vi "Warfortheworlds.vi"() -> ()   [LabVIEW 2021]
panel:
  out "ReadComplete":bool
  out "CountComplete":bool
  out "number":i32
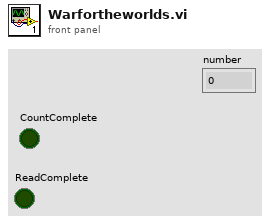
[diagram p1: front panel]
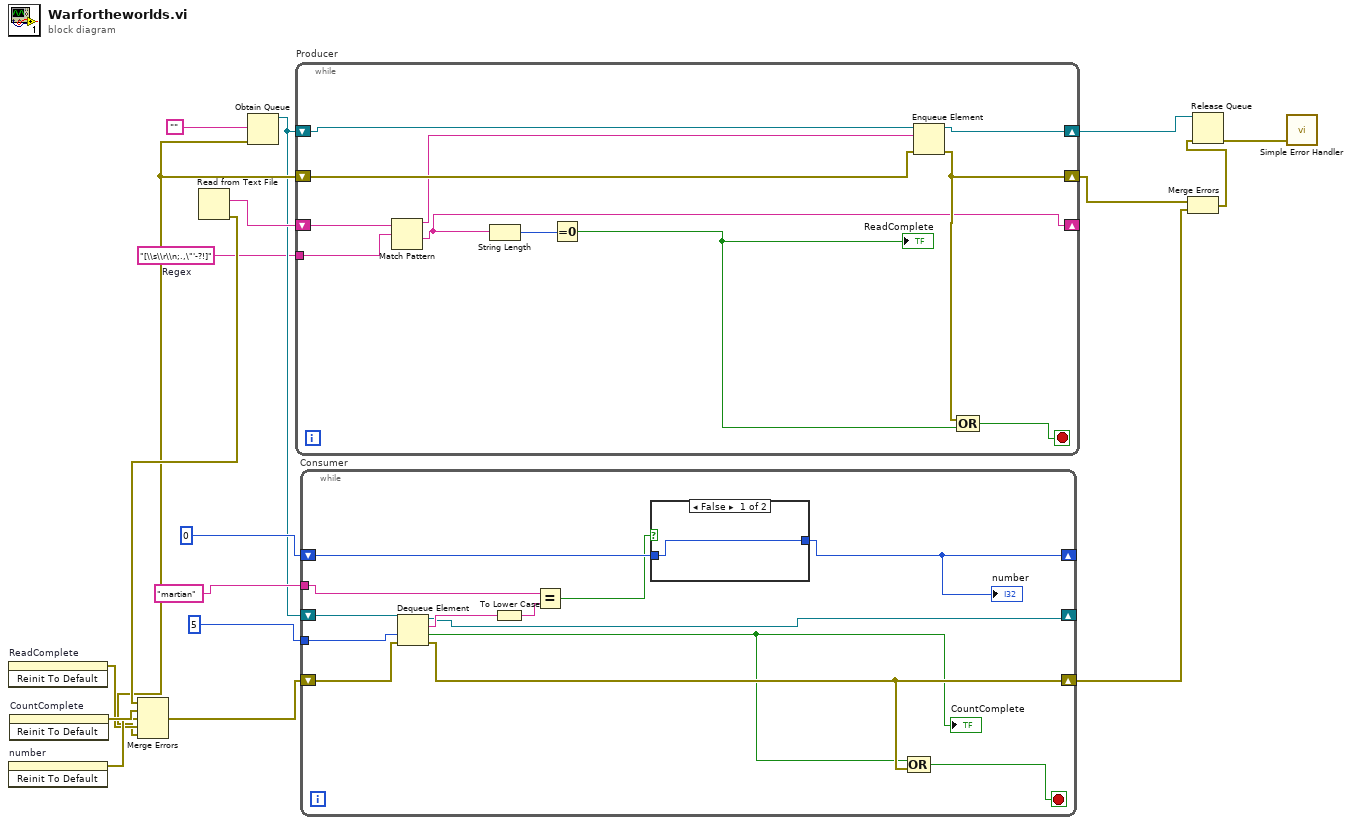
[diagram p0: block diagram]
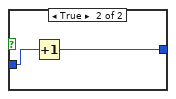
[diagram p2: hidden frame]
diagram:
  w1 = "[\\s\\r\\n;.,\"'-?!]"  # Regex
  n1 = invoke on="ReadComplete" class="Bool (strict)" method="Reinit To Default"() -> (error out=w7:errorcluster)  [unwired: 3 in, 2 out]
  n2 = invoke on="number" class="DigNum (strict)" method="Reinit To Default"() -> (error out=w8:errorcluster)  [unwired: 3 in, 2 out]
  n3 = invoke on="CountComplete" class="Bool (strict)" method="Reinit To Default"() -> (error out=w9:errorcluster)  [unwired: 3 in, 2 out]
  n4 = Read from Text File() -> (text=w17:string, error out=w6:errorcluster)  [unwired: 4 in, 2 out]
  n5 = Obtain Queue(element data type="") -> (queue out=w3:refnum<queue>, error out=w5:errorcluster)  [unwired: 4 in, 1 out]
  n6 = Merge Errors(w6, w9, w8, w7, w5) -> (w4:errorcluster)
  n7 = while "Producer" {
    shift-right: [w27] -> w14
    shift-left: w3 -> [w29]
    shift-right: [w23] -> w15
    shift-left: w5 -> [w28]
    shift-right: [w22] -> _
    shift-left: w17 -> [w26]
    tunnel: w1 -> [w19]
    stop <- w21 stop-if-true
    n8 = Match Pattern(string=w26, regular expression=w19) -> (before substring=w20:string, after substring=w22:string)  [unwired: 1 in, 2 out]
    n9 = String Length(string=w22) -> (length=w25:i32)
    n10 = Equal To 0?(x=w25) -> (x = 0?=w24:bool)
    "ReadComplete" <- w24
    n11 = Enqueue Element(queue=w29, element=w20, error in (no error)=w28) -> (queue out=w27:refnum<queue>, error out=w23:errorcluster)  [unwired: 1 in, 1 out]
    n12 = Compound Arithmetic op=OR(w23, w24) -> (w21:bool)
  }
  n13 = while "Consumer" {
    shift-right: [w32] -> _
    shift-left: 0 -> [w33]
    shift-right: [w31] -> _
    shift-left: w3 -> [w40]
    shift-right: [w39] -> w2
    shift-left: w4 -> [w42]
    tunnel: "martian" -> [w34]
    tunnel: 5 -> [w41]
    stop <- w38 stop-if-true
    n14 = Dequeue Element(queue=w40, timeout in ms (-1)=w41, error in (no error)=w42) -> (queue out=w31:refnum<queue>, element=w35:string, timed out?=w37:bool, error out=w39:errorcluster)
    "CountComplete" <- w37
    n15 = To Lower Case(string=w35) -> (all lower case string=w36:string)
    n16 = Equal?(x=w34, y=w36) -> (x = y?=w30:bool)
    n17 = case shown="False" w30 {
      tunnel: w33 -> [w43 w45]
      tunnel: [w43 w44] -> w32
      frame False {
      }
      frame True {
        n18 = Increment(x=w45) -> (x+1=w44:i32)
      }
    }
    "number" <- w32
    n19 = Compound Arithmetic op=OR(w37, w39) -> (w38:bool)
  }
  n20 = Merge Errors(w15, w2) -> (w16:errorcluster)
  n21 = Release Queue(queue=w14, error in (no error)=w16) -> (error out=w13:errorcluster)  [unwired: 1 in, 2 out]
  n22 = call <vilib>:"Simple Error Handler.vi"("error in (no error)"=w13) -> ()  [unwired: 4 in, 5 out]
